vi "Create NI 9474 - Counter Driven Output.vi"(8 "error in":errorcluster, 10 "drive from slot":T3, 11 "channel settings":T1[](array[typedef])) -> (0 "error out":errorcluster, 3 "NI 9474 out":refnum<class "NI 9474.lvclass">)   [LabVIEW 2020, in "Scan Engine Scripting.lvlib" / "NI 9474.lvclass"]
doc: "Creates and configures an instance of a NI-9474 counter driven output module that can be used to set a slot in a Scan Engine custom device chassis."
uses:
  NI 9474.lvclass
  Mode Classes/Counter Driven Output Mode/Drive from Slot.ctl
  Mode Classes/Controls/counter driven output channel settings.ctl
  Channel Classes/Counter Driven Output Channel/Counter Driven State.ctl
  Mode Classes/Counter Driven Output Mode/Counter Driven Output Mode.lvclass
  C:/jenkins/workspace/ercat-custom-device_release_20.4/Custom Device Source/Scripting/Modules/Mode Classes/Mode/Mode.lvclass
  c3a9027c-5729-4a7d-9244-87c818816035.vi
  Channel Classes/Counter Driven Output Channel/Counter Driven Output Channel.lvclass
  Scan Engine Scripting.lvlib
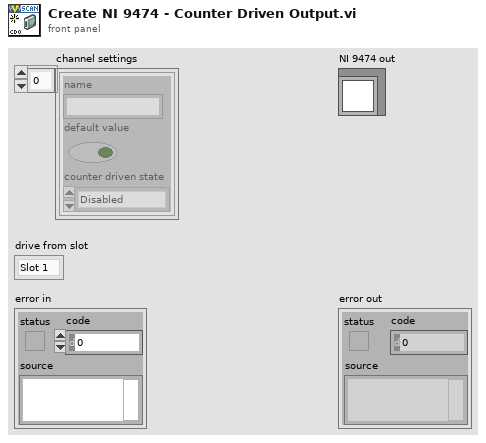
[diagram p1: front panel]
types:
  T1 = typedef "Scan Engine Scripting.lvlib/counter driven output channel settings.ctl" = cluster{"name":string, "default value":bool, "counter driven state":T2}
  T2 = typedef "Scan Engine Scripting.lvlib/Counter Driven Output Channel.lvclass/Counter Driven State.ctl" = enum16{"Disabled", "Enabled"}
  T3 = typedef "Scan Engine Scripting.lvlib/Counter Driven Output Mode.lvclass/Drive from Slot.ctl" = enum16{"Slot 1", "Slot 2", "Slot 3", "Slot 4", "Slot 5", "Slot 6", "Slot 7", "Slot 8"}
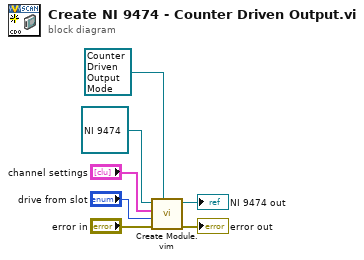
[diagram p0: block diagram]
diagram:
  n1 = call "Create Module.vim"("mode"=refnum<class "Counter Driven Output Mode.lvclass"> refnum ("Scan Engine Scripting.lvlib:Counter Driven Output Mode.lvclass"), "error in"="error in", "mode settings"="drive from slot", "channel settings"="channel settings", "module in"=refnum<class "NI 9474.lvclass"> refnum ("NI 9474 in")) -> ("error out"=→"error out":errorcluster, "module out"=→"NI 9474 out":refnum<class "NI 9474.lvclass">)  [unwired: 5 in]
